vi "Send Request.vi"(8 "error in (no error)":errorcluster, 9 "Parent Message":refnum<class "Message Class.lvclass">, 10 "Message to send":refnum<class "Request Message.lvclass">, 11 "object in":refnum<class "JuPyter_Client.lvclass">) -> (0 "error out":errorcluster, 1 "Reply Back":refnum<class "Reply Message.lvclass">, 2 "Message Out":refnum<class "Request Message.lvclass">, 3 "object out":refnum<class "JuPyter_Client.lvclass">)   [LabVIEW 2018, in "JuPyter_Client.lvclass"]
doc: "Prepare and send a request message"
uses:
  JuPyter_Client.lvclass
  Base Classes/Request Message/Request Message.lvclass
  C:/Users/gavin/Documents/LabVIEW Data/LabVIEW-Bits/Connectivity/Jupyter Client/Base Classes/Message Class/Message Class.lvclass
  Base Classes/Message Class/Message Class.lvclass
  Base Classes/Reply Message/Reply Message.lvclass
  JuPyter_Client.lvclass/JuPyter_Client.ctl
  Base Classes/Message Class/protected/header_dict.ctl
  SHA256/SHA256.lvlib
  <vilib>/addons/zeromq/zmq_socket.lvclass
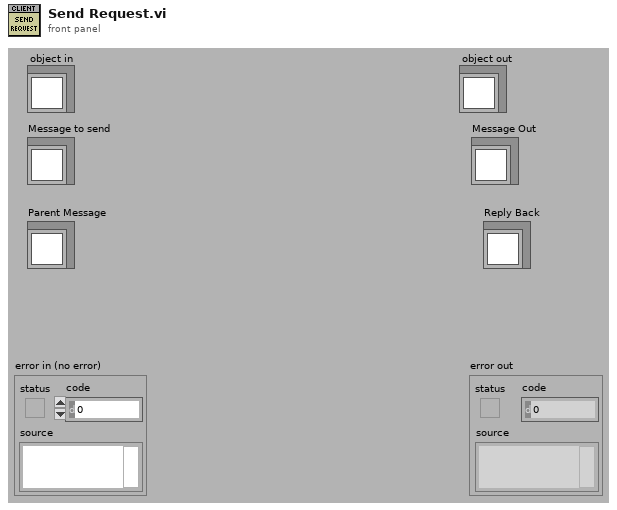
[diagram p1: front panel]
types:
  T1 = typedef "ClientMessaging.lvlib/Message Class.lvclass/header_dict.ctl" = cluster{"msg_id":string, "username":string, "session":string, "date":timestamp, "msg_type":string, "version":string}
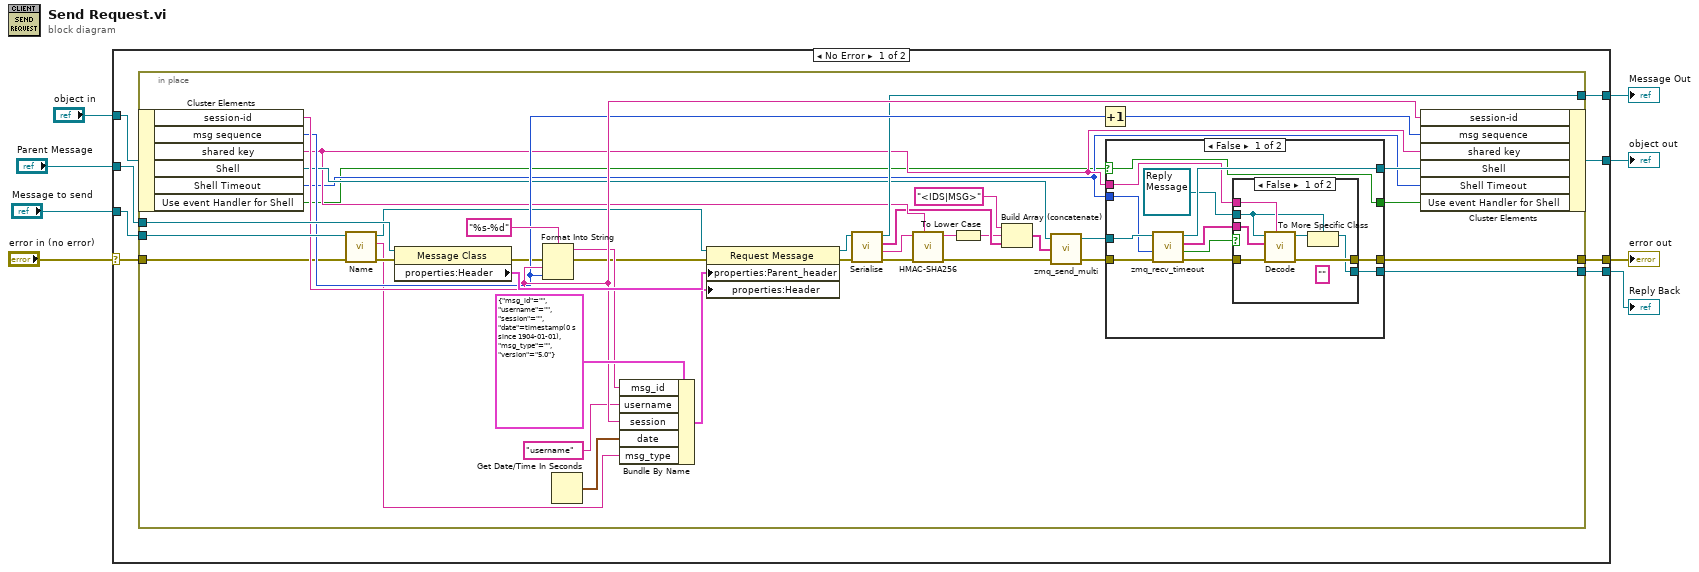
[diagram p0: block diagram]
diagram:
  n1 = case shown="No Error" "error in (no error)" {
    selector: "error in (no error)" -> [w14 w82]
    tunnel: [w9 w82] -> w6
    tunnel: [w15 w81] -> w5
    tunnel: "object in" -> [w16 w81]
    tunnel: "Parent Message" -> [w13 _]
    tunnel: "Message to send" -> [w12 w80]
    tunnel: [w11 w80] -> w2
    tunnel: [w10 _] -> w1
    frame No Error {
      n2 = in-place {
        in-place-border: w14 -> [w36]
        in-place-border: w13 -> [w55]
        in-place-border: w12 -> [w54]
        in-place-border: [w40] -> w11
        in-place-border: [w28] -> w10
        in-place-border: [w30] -> w9
        n3 = in-place-cluster #1(w16) -> ("session-id"=w47:string, "msg sequence"=w46:u64, "shared key"=w29:string, "Shell"=w34:refnum<class "zmq_socket.lvclass">, "Shell Timeout"=w19:i32, "Use event Handler for Shell"=w18:bool)
        n4 = call-dynamic "Name.vi"("error in (no error)"=w36, "object in"=w54) -> ("error out"=w35:errorcluster, "Name"=w27:string, "object out"=w37:refnum<class "Request Message.lvclass">)  [unwired: 7 in]
        n5 = property class="Message Class"(reference=w55, error in=w35) -> (error out=w43:errorcluster, "properties:Header"=w53:T1)  [unwired: 1 out]
        n6 = Format Into String(format string="%s-%d", error in=w43, w47, w46) -> (resulting string=w44:string, error out=w42:errorcluster)  [unwired: 1 in]
        n7 = Get Date/Time In Seconds() -> (seconds since 1Jan1904=w49:timestamp)
        n8 = Bundle By Name(cluster=T1 {"msg_id"="", "username"="", "session"="", "date"=timestamp(0 s since 1904-01-01), "msg_type"="", "version"="5.0"} ("Header"), "msg_id"=w44, "username"="username", "session"=w47, "date"=w49, "msg_type"=w27) -> (w50:T1)
        n9 = property class="Request Message"(reference=w37, error in=w42, "properties:Parent_header"=w53, "properties:Header"=w50) -> (reference out=w52:refnum<class "Request Message.lvclass">, error out=w41:errorcluster)
        n10 = call-dynamic "Serialise.vi"("error in (no error)"=w41, "object in"=w52) -> ("error out"=w39:errorcluster, 1:"Serialised String"=w23:string, 2:"Serialised String"=w22:string[], "object out"=w40:refnum<class "Request Message.lvclass">)  [unwired: 6 in]
        n11 = call <vilib>:"HMAC-SHA256.vi"("Key"=w29, "error In"=w39, "String to Encode"=w23) -> ("error Out"=w26:errorcluster, "Hash String"=w24:string)  [unwired: 7 in]
        n12 = To Lower Case(string=w24) -> (all lower case string=w20:string)
        n13 = Build Array (concatenate)("<IDS|MSG>", w20, w22) -> (w21:string[])
        n14 = call <vilib>:"zmq_send_multi.vi"("error in"=w26, "parts"=w21, "socket in"=w34) -> ("error out"=w32:errorcluster, "socket out"=w33:refnum<class "zmq_socket.lvclass">)  [unwired: 1 in]
        n15 = Increment(x=w46) -> (x+1=w45:u64)
        n16 = case shown="False" w18 {
          selector: w18 -> [w56 w77]
          tunnel: w33 -> [w67 w79]
          tunnel: w32 -> [w66 w78]
          tunnel: [w65 w79] -> w31
          tunnel: [w62 w78] -> w30
          tunnel: w29 -> [w61 _]
          tunnel: [w60 _] -> w28
          tunnel: w19 -> [w57 _]
          tunnel: [w56 w77] -> w17
          frame False {
            n17 = call <vilib>:"zmq_recv_timeout.vi"("error in"=w66, "timeout (ms)"=w57, "socket in"=w67) -> ("error out"=w63:errorcluster, "timeout?"=w58:bool, "parts"=w64:string[], "socket out"=w65:refnum<class "zmq_socket.lvclass">)  [unwired: 1 in]
            n18 = case shown="False" w58 {
              tunnel: w64 -> [w68 _]
              tunnel: w63 -> [w73 w75]
              tunnel: [w72 w75] -> w62
              tunnel: w61 -> [w71 _]
              tunnel: [w70 w76] -> w60
              tunnel: refnum<class "Reply Message.lvclass"> refnum ("Reply Back") -> [w69 w76]
              frame False {
                (unwired) "" ("delimiter (Tab)")
                n19 = call "Decode.vi"("Session Key"=w71, "error in (no error)"=w73, "Message In"=w68, "object in"=w69) -> ("error out"=w72:errorcluster, "object out"=w74:refnum<class "Message Class.lvclass">)  [unwired: 3 in, 3 out]
                n20 = To More Specific Class(target class=w69, reference=w74) -> (specific class reference=w70:refnum<class "Reply Message.lvclass">)  [unwired: 1 in, 1 out]
              }
              frame True {
              }
            }
          }
          frame True {
          }
        }
        n21 = in-place-cluster #1("session-id"=w47, "msg sequence"=w45, "shared key"=w29, "Shell"=w31, "Shell Timeout"=w19, "Use event Handler for Shell"=w17) -> (w15:refnum<class "JuPyter_Client.lvclass">)
      }
    }
    frame Error {
    }
  }
  "error out" <- w6
  "object out" <- w5
  "Message Out" <- w2
  "Reply Back" <- w1
